vi "Aux CO2 Set LoFlo Compensation.vi"(8 "error In":errorcluster, 10 "Baro Pressure":u32=760, 11 "Serial Port In":T1={"termination char"=10, "End read on termination character?"=TRUE, "Enabled?"=FALSE, "VISA resource name"="COM1", "baud rate"=9600, "data bits"=8, "parity"=enum."None", "stop bits"=10, "flow control"=0, "timeout (ms)"=10000, "Input buffer size"=4096, "End write on termination character?"=TRUE, "XON Char"=17, "XOFF Char"=19} {"XOFF Char" format="%.0x"; "XON Char" format="%.0x"; "flow control" items=["None"=0, "XON/XOFF"=1, "RTS/CTS"=2, "DTR/DSR"=4]; "stop bits" items=["1.0"=10, "1.5"=15, "2.0"=20]; "data bits" min=5 max=8 step=1; "baud rate" items=["75"=75, "110"=110, "134"=134, "150"=150, "300"=300, "600"=600, "1200"=1200, "1800"=1800, "2400"=2400, "4800"=4800, "7200"=7200, "9600"=9600, "14400"=14400, "19200"=19200, "28800"=28800, "38400"=38400, "56000"=56000, "57600"=57600, "115200"=115200, "128000"=128000, "230400"=230400]; "termination char" format="%.0x"}) -> (0 "error Out":errorcluster, 3 "Serial Port Out":T1={"termination char"=10, "End read on termination character?"=TRUE, "Enabled?"=TRUE, "VISA resource name"="COM1", "baud rate"=9600, "data bits"=8, "parity"=enum."None", "stop bits"=10, "flow control"=0, "timeout (ms)"=10000, "Input buffer size"=4096, "End write on termination character?"=FALSE, "XON Char"=17, "XOFF Char"=19} {"XOFF Char" format="%.0x"; "XON Char" format="%.0x"; "flow control" items=["None"=0, "XON/XOFF"=1, "RTS/CTS"=2, "DTR/DSR"=4]; "stop bits" items=["1.0"=10, "1.5"=15, "2.0"=20]; "baud rate" items=["1.0"=10, "1.5"=15, "2.0"=20]; "termination char" format="%.0x"})   [LabVIEW 2016]
uses:
  Controls/Serial Visa Control.ctl
  Controls/SerialPortControl.ctl
panel:
  out "appended array":u32[](array[numeric]) format="%x"
  out "x-1":u32 format="%x"
  out "Baro string":string
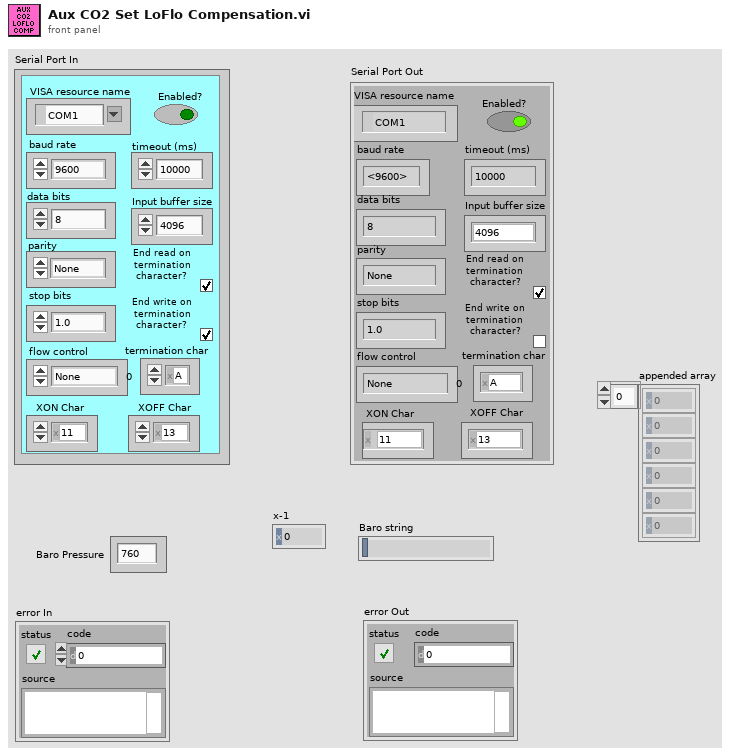
[diagram p1: front panel]
types:
  T1 = typedef "Serial Visa Control.ctl" = cluster{"termination char":u8, "End read on termination character?":bool, "Enabled?":bool, "VISA resource name":refnum<visa-resource-name>, "baud rate":u32, "data bits":u16, "parity":enum16{"None", "Odd", "Even", "Mark", "Space"}, "stop bits":u16, "flow control":u16, "timeout (ms)":u32, "Input buffer size":u32, "End write on termination character?":bool, "XON Char":u8, "XOFF Char":u8}
  T2 = typedef "SerialPortControl.ctl" = enum16{"Initialize", "Write Data", "Read Data", "Close Port"}
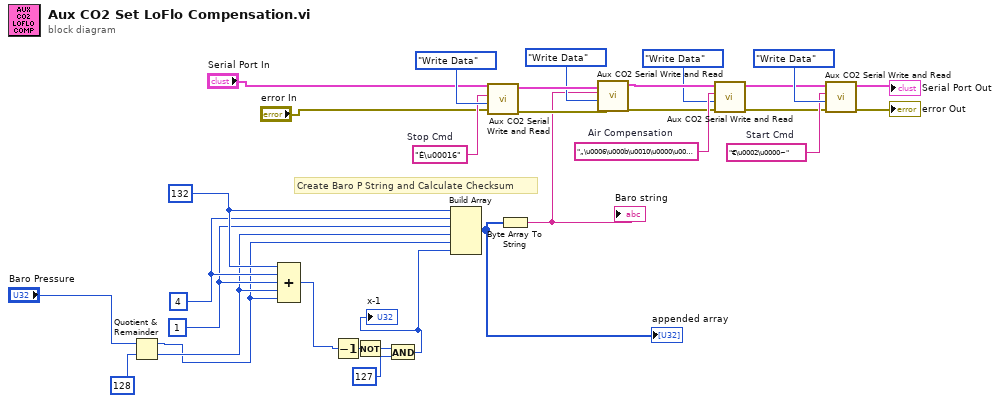
[diagram p0: block diagram]
diagram:
  w5 = "€\u0002\u0000~"  # Start Cmd
  w23 = "É\u00016"  # Stop Cmd
  w22 = "„\u0006\u000b\u0010\u0000\u0000\u0000["  # Air Compensation
  w10 = 1
  w11 = 4
  w12 = 132
  # "Create Baro P String and Calculate Checksum"
  n1 = Quotient & Remainder(x="Baro Pressure", y=u32 128) -> (x-y*floor(x/y)=w8:u32, floor(x/y)=w9:u32)
  n2 = Compound Arithmetic op=ADD(w12, w11, w10, w9, w8) -> (w7:u32)
  n3 = Decrement(x=w7) -> (x-1=w30:u32)
  n4 = Not(x=w30) -> (.not. x?=w14:u32)
  n5 = And(x=w14, y=127) -> (x .and. y?=w13:u32)
  "x-1" <- w13
  n6 = Build Array(w12, w11, w10, w9, w8, w13) -> (w28:u32[])
  "appended array" <- w28
  n7 = call "Aux CO2 Serial Write and Read.vi"("error in"="error In", "Action"=SerialPortControl."Write Data", "string to write"=w23, "Serial Port"="Serial Port In") -> ("error IO"=w26:errorcluster, "Serial Port Out"=w25:T1)  [unwired: 2 out]
  n8 = Byte Array To String(unsigned byte array=w28) -> (string=w17:string)
  "Baro string" <- w17
  n9 = call "Aux CO2 Serial Write and Read.vi"("error in"=w26, "Action"=SerialPortControl."Write Data", "string to write"=w17, "Serial Port"=w25) -> ("error IO"=w20:errorcluster, "Serial Port Out"=w21:T1)  [unwired: 2 out]
  n10 = call "Aux CO2 Serial Write and Read.vi"("error in"=w20, "Action"=SerialPortControl."Write Data", "string to write"=w22, "Serial Port"=w21) -> ("error IO"=w3:errorcluster, "Serial Port Out"=w4:T1)  [unwired: 2 out]
  n11 = call "Aux CO2 Serial Write and Read.vi"("error in"=w3, "Action"=SerialPortControl."Write Data", "string to write"=w5, "Serial Port"=w4) -> ("error IO"=→"error Out":errorcluster, "Serial Port Out"=→"Serial Port Out":T1)  [unwired: 2 out]
